vi "Git Branch.vi"(8 "error in (no error)":errorcluster, 11 "Git in":refnum<class "Git.lvclass">) -> (0 "error out":errorcluster, 1 "all branches":string[](array[string]), 2 "active branch":string, 3 "Git out":refnum<class "Git.lvclass">)   [LabVIEW 2019, in "Git.lvclass"]
uses:
  Git.lvclass
  Typedefs/Commands.git--combo.ctl
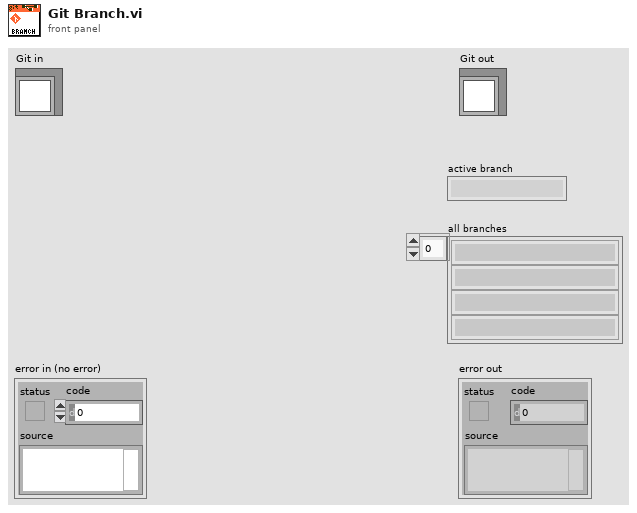
[diagram p1: front panel]
types:
  T1 = typedef "Git.lvclass/Commands.git--combo.ctl" = string
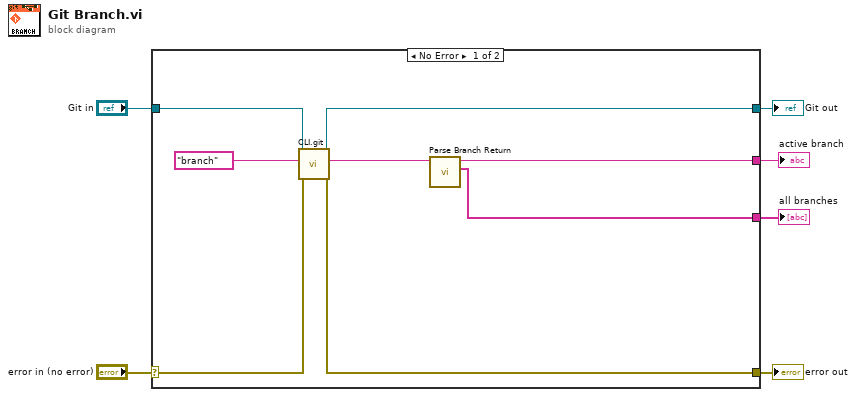
[diagram p0: block diagram]
diagram:
  n1 = case shown="No Error" "error in (no error)" {
    selector: "error in (no error)" -> [w14 w16]
    tunnel: [w13 w16] -> w5
    tunnel: [w12 w15] -> w3
    tunnel: "Git in" -> [w11 w15]
    tunnel: [w8 _] -> w2
    tunnel: [w7 _] -> w1
    frame No Error {
      n2 = call "CLI.git.vi"("error in (no error)"=w14, "Command"=T1 "branch", "Git in"=w11) -> ("error out"=w13:errorcluster, "standard output"=w9:string, "Git out"=w12:refnum<class "Git.lvclass">)  [unwired: 4 in, 2 out]
      n3 = call "Parse Branch Return.vi"("standard output"=w9) -> ("branches"=w7:string[], "active branch"=w8:string)  [unwired: 9 in]
    }
    frame Error {
    }
  }
  "error out" <- w5
  "Git out" <- w3
  "active branch" <- w2
  "all branches" <- w1
